vi "Get measurementservice_DMMVoltageRequest.vi"(8 "error in (no error)":errorcluster, 11 "gRPCid":T2) -> (0 "error out":errorcluster, 2 "Message Data":T1, 3 "gRPCid out":T2)   [LabVIEW 2019, in "HVC.lvlib" / "HVC.lvclass"]
uses:
  HVC.lvclass
  gRPC lvSupport/Server API/typeDefs/grpcId.ctl
  measurementservice_DMMVoltageRequest_Data.ctl
  a51dd2a7-b5c1-4c09-9df4-8cd9d3bd0c19.vi
  gRPC lvSupport/Server API/Server/Get Server DLL Path.vi
  gRPC lvSupport/gprc-lvsupport.lvlib
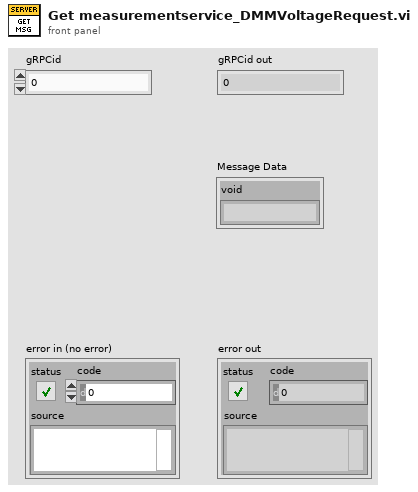
[diagram p1: front panel]
types:
  T1 = typedef "HVC.lvlib/HVC.lvclass/measurementservice_DMMVoltageRequest_Data.ctl" = cluster{"void":string}
  T2 = typedef "HVC.lvlib/gprc-lvsupport.lvlib/grpcId.ctl" = u64
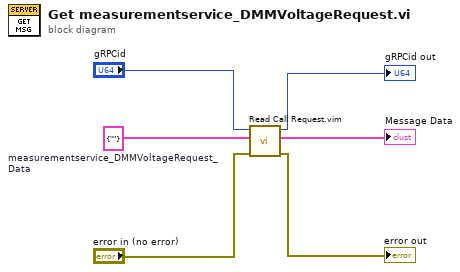
[diagram p0: block diagram]
diagram:
  w2 = T1 {"void"=""}  # measurementservice_DMMVoltageRequest_Data
  n1 = call "Read Call Request.vim"("error in (no error)"="error in (no error)", "Data Type"=w2, "gRPCid in"="gRPCid") -> ("error out"=→"error out":errorcluster, "Request Data"=→"Message Data":T1, "gRPCid out"=→"gRPCid out":T2)  [unwired: 6 in]
